vi "_TreeItem.Property.Get.Dictionary.vi"(8 "error in (no error)":errorcluster, 11 "DictionaryProperty":refnum<k24>) -> (0 "error out":errorcluster, 2 "Dictionary Variant":variant, 3 "DictionaryProperty out":refnum<k24>)   [LabVIEW 2016, in "Advanced System Definition.lvlib"]
uses:
  SysDef API/Advanced System Definition.lvlib
  NationalInstruments.VeriStand.SystemStorage
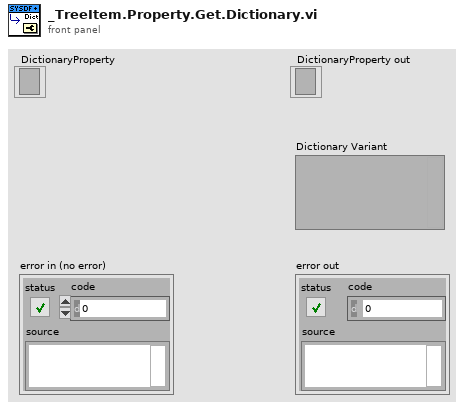
[diagram p1: front panel]
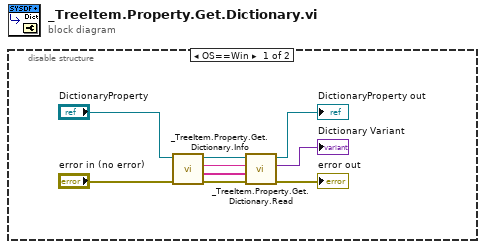
[diagram p0: block diagram]
diagram:
  n1 = disable-structure shown="OS==Win" {
    frame condition #0 (active) {
      n2 = call "_TreeItem.Property.Get.Dictionary.Info.vi"("error in (no error)"="error in (no error)", "DictionaryProperty"="DictionaryProperty") -> ("error out"=w7:errorcluster, "Keys"=w4:string[], "DictionaryType"=w5:string, "DictionaryProperty out"=w6:refnum<k24>)  [unwired: 6 in]
      n3 = call "_TreeItem.Property.Get.Dictionary.Read.vi"("error in (no error)"=w7, "Keys"=w4, "Type"=w5, "DictionaryProperty"=w6) -> ("error out"=→"error out":errorcluster, "Dictionary Variant"=→"Dictionary Variant":variant, "DictionaryProperty out"=→"DictionaryProperty out":refnum<k24>)  [unwired: 5 in]
    }
    frame condition #1 {
    }
  }
